vi "Program_1_Sine_Wave.vi"() -> ()   [LabVIEW 2015]
uses:
  <vilib>/measure/maspectr.llb/FFT Spectrum (Mag-Phase) for 1 Chan.vi
  <vilib>/measure/NI_MABase.lvlib
  <vilib>/measure/NI_MAPro.lvlib
panel:
  out "FFT Amplitude":cluster{"f0":dbl, "df":dbl, "magnitude":dbl[]}(graph)
  out "Sine Wave":waveform(dbl)(graph)={"t0"=timestamp(0 s since 1904-01-01), "dt"=0.0005, "Y"=array[1000 elements]}
  in  "sampling info":cluster{"Fs":dbl, "#s":dbl}={"Fs"=2000.0, "#s"=1000.0} {"Fs" format="%.2p"}
  in  "signal type":T1(ring)
  in  "phase":dbl format="%.2p"
  in  "amplitude":dbl=5.0 format="%0.2p"
  in  "frequency":dbl=4.0 format="%0.2p"
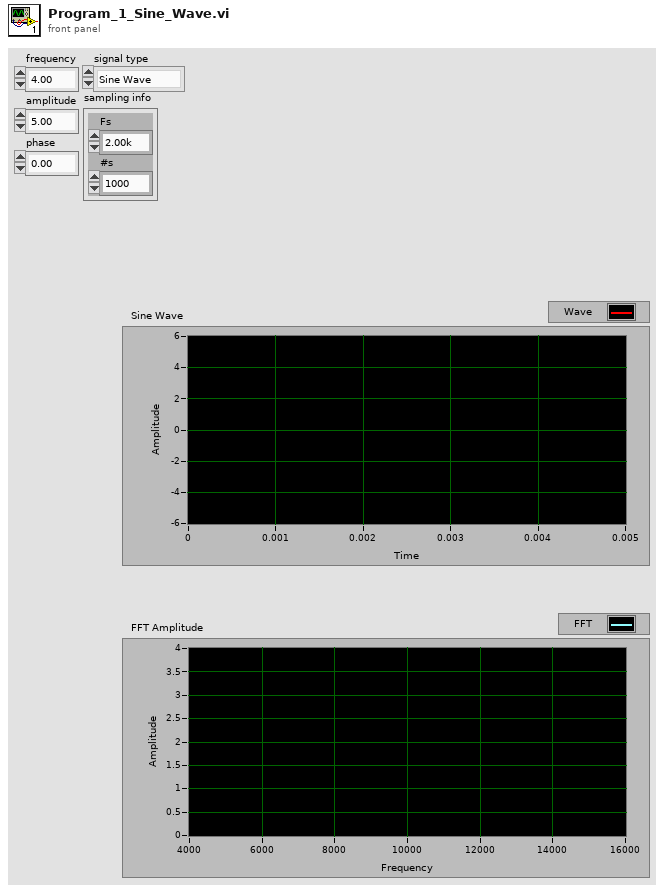
[diagram p1: front panel]
types:
  T1 = enum16{"Sine Wave", "Triangle Wave", "Square Wave", "Sawtooth Wave"}
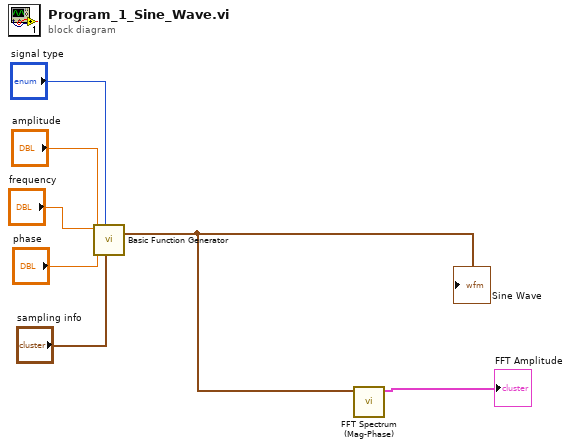
[diagram p0: block diagram]
diagram:
  n1 = call <vilib>:"Basic Function Generator.vi"("sampling info"="sampling info", "signal type"="signal type", "phase"="phase", "amplitude"="amplitude", "frequency"="frequency") -> ("signal out"=w2:waveform(dbl))  [unwired: 4 in, 2 out]
  "Sine Wave" <- w2
  n2 = call-poly <vilib>:"FFT Spectrum (Mag-Phase).vi"("time signal"=w2) -> ("magnitude"=→"FFT Amplitude":cluster{"f0":dbl, "df":dbl, "magnitude":dbl[]})  [unwired: 6 in, 4 out]
